vi "globalFileNeologist.vi"(9 "FileNeologist in":refnum<class "FileNeologist.lvclass">, 10 "Action":enum16{"Write", "Read"}(ring)) -> (1 "FileNeologist out":refnum<class "FileNeologist.lvclass">)   [LabVIEW 2011, in "Tools.lvlib" / "Filing.lvlib"]
doc: "Makes the FileNeologist object global, such that all objects using it has the most current state."
uses:
  Filing.lvlib
  FileNeologist.lvclass
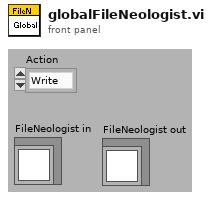
[diagram p1: front panel]
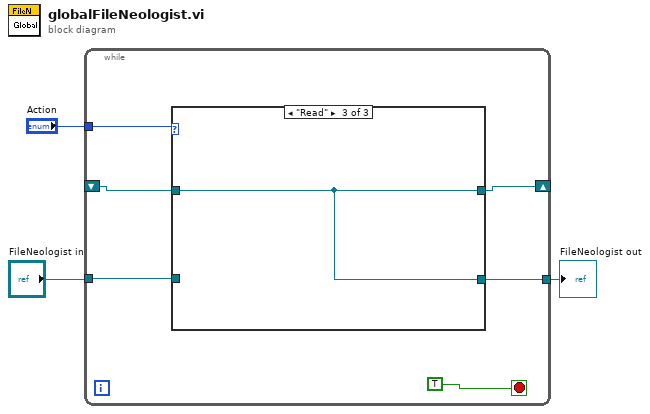
[diagram p0: block diagram]
diagram:
  n1 = while {
    tunnel: "Action" -> [w9]
    shift-right: [w4] -> _
    shift-left: _ -> [w6]
    tunnel: "FileNeologist in" -> [w7]
    tunnel: [w5] -> w1
    stop <- TRUE stop-if-true
    n2 = case shown="\"Read\"" w9 {
      tunnel: [w11 w12 w13] -> w4
      tunnel: w7 -> [w10 w12 _]
      tunnel: w6 -> [w11 _ w13]
      tunnel: [w10 w12 w13] -> w5
      frame Default {
      }
      frame "Write" {
      }
      frame "Read" {
      }
    }
  }
  "FileNeologist out" <- w1
